vi "AlliGator Update Settings Decay Shift Parameters Visibility.vi"(8 "error in":errorcluster, 11 "Shift Parameters Refnum":refnum<vi>) -> (0 "error out":errorcluster, 3 "Shift Parameters Refnum":refnum<vi>)   [LabVIEW 2021, in "AlliGator Settings.lvlib"]
doc: "Updates the visibility of controls related to shift pre-processing operations."
uses:
  AlliGator Settings.lvlib
panel:
  # "see the AlliGator License on the block diagram (Ctrl+E or Window:Show Block Diagram)"
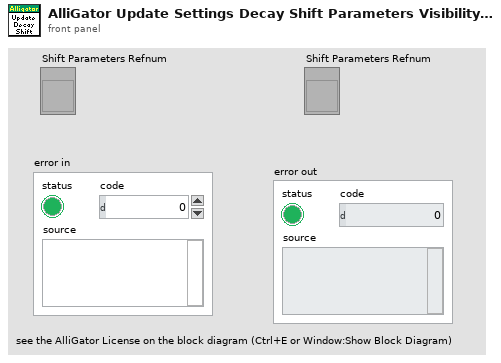
[diagram p1: front panel]
types:
  T1 = typedef "IRF Analysis Parameters.ctl" = cluster{"Type":T2, "Shift":dbl[unit], "Threshold":dbl, "Rotate":bool}
  T2 = typedef "IRF Analysis Method.ctl" = enum16{"Default", "CFD", "Threshold", "Cross-Correlation"}
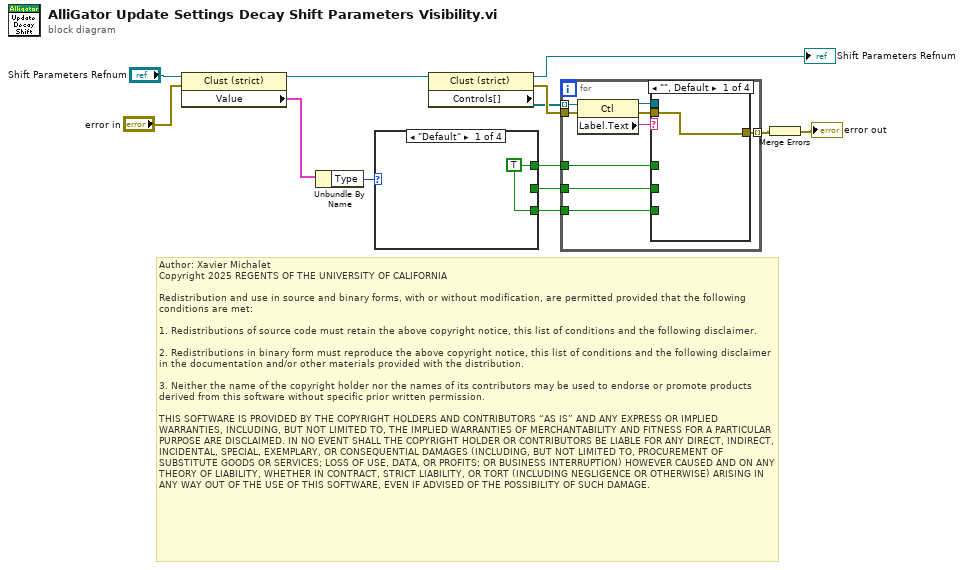
[diagram p0: block diagram]
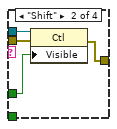
[diagram p2: hidden frame]
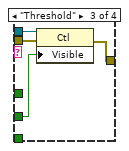
[diagram p3: hidden frame]
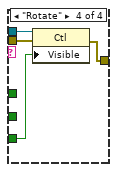
[diagram p4: hidden frame]
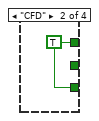
[diagram p5: hidden frame]
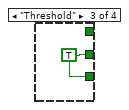
[diagram p6: hidden frame]
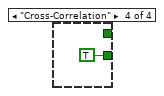
[diagram p7: hidden frame]
diagram:
  # "Author: Xavier Michalet\nCopyright 2025 REGENTS OF THE UNIVERSITY OF CALIFORNIA\n\nRedistribution and use in source and binary forms, with or without modification, are permitted provided that the following conditions are met:\n\n1. Redistributions of source code must retain the above copyright notice, this list of conditions and the following disclaimer.\n\n2. Redistributions in binary form must reproduce the above copyright notice, this list of conditions and the following disclaimer in the documentation and/or other materials provided with the distribution.\n\n3. Neither the name of the copyright holder nor the names of its contributors may be used to endorse or promote products derived from this software without specific prior written permission.\n\nTHIS SOFTWARE IS PROVIDED BY THE COPYRIGHT HOLDERS AND CONTRIBUTORS “AS IS” AND ANY EXPRESS OR IMPLIED WARRANTIES, INCLUDING, BUT NOT LIMITED TO, THE IMPLIED WARRANTIES OF MERCHANTABILITY AND FITNESS FOR A PARTICULAR PURPOSE ARE DISCLAIMED. IN NO EVENT SHALL THE COPYRIGHT HOLDER OR CONTRIBUTORS BE LIABLE FOR ANY DIRECT, INDIRECT, INCIDENTAL, SPECIAL, EXEMPLARY, OR CONSEQUENTIAL DAMAGES (INCLUDING, BUT NOT LIMITED TO, PROCUREMENT OF SUBSTITUTE GOODS OR SERVICES; LOSS OF USE, DATA, OR PROFITS; OR BUSINESS INTERRUPTION) HOWEVER CAUSED AND ON ANY THEORY OF LIABILITY, WHETHER IN CONTRACT, STRICT LIABILITY, OR TORT (INCLUDING NEGLIGENCE OR OTHERWISE) ARISING IN ANY WAY OUT OF THE USE OF THIS SOFTWARE, EVEN IF ADVISED OF THE POSSIBILITY OF SUCH DAMAGE."
  n1 = property class="Clust (strict)"(reference="Shift Parameters Refnum", error in="error in") -> (reference out=w3:refnum<vi>, "Value"=w2:T1)  [unwired: 1 out]
  n2 = Unbundle By Name(w2) -> ("Type"=w4:T2)
  n3 = case shown="\"Default\"" w4 {
    tunnel: [_ _ w16 _] -> w9
    tunnel: [w14 w15 _ _] -> w8
    tunnel: [w14 w15 w16 TRUE ("Visible")] -> w10
    frame "Default" {
      w14 = TRUE ("Visible")
    }
    frame "CFD" {
      w15 = TRUE ("Visible")
    }
    frame "Threshold" {
      w16 = TRUE ("Visible")
    }
    frame "Cross-Correlation" {
    }
  }
  n4 = property class="Clust (strict)"(reference=w3) -> (reference out=→"Shift Parameters Refnum":refnum<vi>, error out=w11:errorcluster, "Controls[]"=w7:refnum<vi>[])  [unwired: 1 in]
  n5 = for {
    tunnel: w7 -> [w26] mode=indexing
    tunnel: w8 -> [w23]
    tunnel: w9 -> [w22]
    tunnel: w10 -> [w21]
    tunnel: w11 -> [w20]
    tunnel: [w18] -> w12 mode=indexing
    n6 = property class="Ctl"(reference=w26, error in=w20) -> (reference out=w24:refnum<vi>, error out=w19:errorcluster, "Label.Text"=w25:string)
    n7 = case shown="\"\", Default" w25 {
      tunnel: w24 -> [_ w31 w35 w39]
      tunnel: w23 -> [_ w30 _ _]
      tunnel: w22 -> [_ _ w34 _]
      tunnel: w21 -> [_ _ _ w38]
      tunnel: w19 -> [w27 w29 w33 w37]
      tunnel: [w27 w28 w32 w36] -> w18
      frame "", Default {
      }
      frame "Shift" {
        n8 = property class="Ctl"(reference=w31, error in=w29, "Visible"=w30) -> (error out=w28:errorcluster)  [unwired: 1 out]
      }
      frame "Threshold" {
        n9 = property class="Ctl"(reference=w35, error in=w33, "Visible"=w34) -> (error out=w32:errorcluster)  [unwired: 1 out]
      }
      frame "Rotate" {
        n10 = property class="Ctl"(reference=w39, error in=w37, "Visible"=w38) -> (error out=w36:errorcluster)  [unwired: 1 out]
      }
    }
  }
  n11 = Merge Errors(w12) -> (→"error out":errorcluster)
